vi "Populate ring controls.vi"(8 "error in (no error)":errorcluster, 9 "Worksheets names":string[](array[string]), 11 "Array":refnum<vi>[](array[refnum])) -> (0 "error out (no error)":errorcluster)   [LabVIEW 2019]
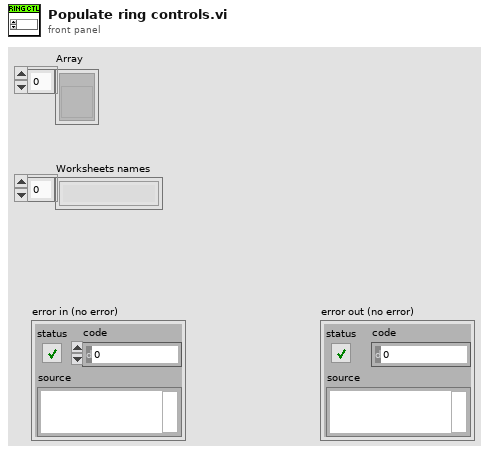
[diagram p1: front panel]
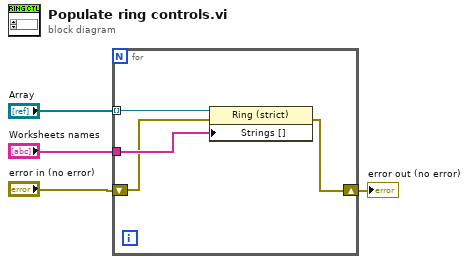
[diagram p0: block diagram]
diagram:
  n1 = for {
    tunnel: "Array" -> [w8] mode=indexing
    tunnel: "Worksheets names" -> [w7]
    shift-right: [w5] -> w1
    shift-left: "error in (no error)" -> [w6]
    n2 = property on="Property Node" class="Ring (strict)"(reference=w8, error in=w6, "Strings []"=w7) -> (error out=w5:errorcluster)  [unwired: 1 out]
  }
  "error out (no error)" <- w1
